vi "New JSON Object (Single String).vi"(7 "key":string, 8 "error in (no error)":errorcluster, 10 "value":string) -> (0 "error out":errorcluster, 3 "JSON Object out":refnum<class "JSON Helper.lvclass">)   [LabVIEW 2016, in "JSON Helper.lvclass"]
doc: "Create a new JSON Object initialized with the given key value pair."
uses:
  JSON Helper/JSON Helper.lvclass
  JSON Object.lvclass
  Insert Key Value Pair (Single String).vi
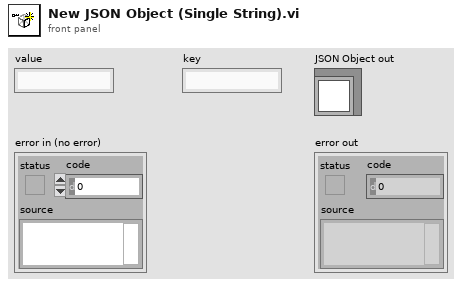
[diagram p1: front panel]
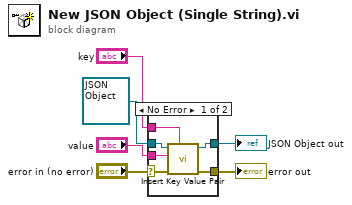
[diagram p0: block diagram]
diagram:
  n1 = case shown="No Error" "error in (no error)" {
    selector: "error in (no error)" -> [w12 w14]
    tunnel: [w11 w14] -> w5
    tunnel: [w9 w13] -> w4
    tunnel: refnum<class "JSON Object.lvclass"> refnum ("JSON Object.lvclass") -> [w10 w13]
    tunnel: "key" -> [w8 _]
    tunnel: "value" -> [w7 _]
    frame No Error {
      n2 = call-poly "Insert Key Value Pair.vi"("key"=w8, "error in (no error)"=w12, "value"=w7, "JSON Object in"=w10) -> ("error out"=w11:errorcluster, "JSON Object out"=w9:refnum<class "JSON Helper.lvclass">)  [unwired: 5 in, 1 out]
    }
    frame Error {
    }
  }
  "error out" <- w5
  "JSON Object out" <- w4
